vi "Set_DO.vi"(0 "reference in":refnum<class "DO.lvclass">, 5 "DO":bool, 11 "error in (no error)":errorcluster) -> (4 "reference out":refnum<class "DO.lvclass">, 15 "error out":errorcluster)   [LabVIEW 2019, in "DO.lvclass"]
uses:
  DO.lvclass
  D:/GIT H4000/H4000/src/Proccess_class/Proccess.lvclass
  DO.lvclass/DO.ctl
  Proccess_class/Proccess.lvclass/Proccess.ctl
  Proccess_class/GetNames.vi
  Proccess_class/GetLogger.vi
  Logger_class/WriteEvent.vi
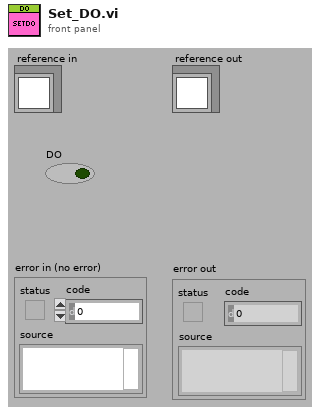
[diagram p1: front panel]
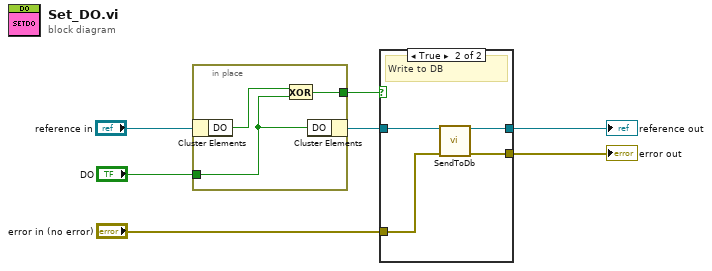
[diagram p0: block diagram]
diagram:
  n1 = in-place {
    in-place-border: "DO" -> [w10]
    in-place-border: [w9] -> w2
    n2 = in-place-cluster #1("reference in") -> ("DO"=w8:bool)
    n3 = Exclusive Or(1:w10, 2:w8) -> (0:w9:bool)
    n4 = in-place-cluster #1("DO"=w10) -> (w1:refnum<class "DO.lvclass">)
  }
  n5 = case shown="True" w2 {
    tunnel: w1 -> [w12 w14]
    tunnel: [w12 w16] -> w4
    tunnel: "error in (no error)" -> [w11 w13]
    tunnel: [w11 w15] -> w6
    frame False {
    }
    frame True {
      # "Write to DB"
      n6 = call "SendToDb.vi"("reference in"=w14, "error in (no error)"=w13) -> ("reference out"=w16:refnum<class "DO.lvclass">, "error out"=w15:errorcluster)  [unwired: 12 in]
    }
  }
  "error out" <- w6
  "reference out" <- w4
